vi "AFscanFineRange.vi"(8 "error in (no error)":errorcluster, 9 "ImageIn":T1, 10 "Session In":T2, 11 "controller in":refnum<k24>) -> (0 "error out":errorcluster, 1 "Image Out":T1, 2 "Session Out":T2, 3 "controller out":refnum<k24>, 4 "MaxVal":dbl, 5 "BestZ":dbl)   [LabVIEW 2019]
uses:
  C:/Users/TTUHEP/Documents/LabVIEW/Other Models/2010/Bin/Aerotech.A3200.dll
  Other Models/2010/Bin/Aerotech.A3200.dll
  <vilib>/vision/Image Controls.llb/IMAQ Image.ctl
  <vilib>/userDefined/High Color/IMAQdx.ctl
  <vilib>/vision/NI_Vision_Development_Module.lvlib
  <vilib>/vision/driver/NI_Vision_Acquisition_Software.lvlib
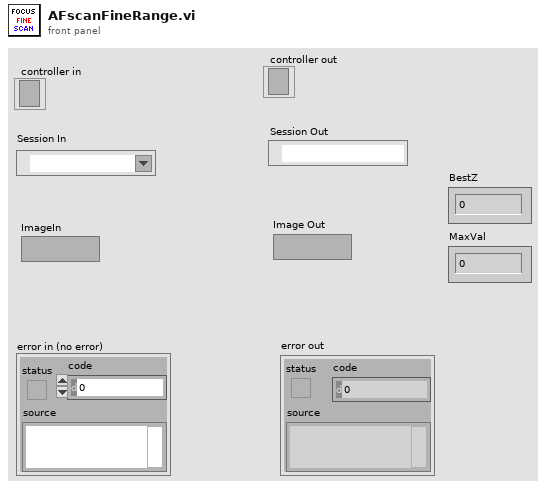
[diagram p1: front panel]
types:
  T1 = typedef "IMAQ Image.ctl" = refnum<image>
  T2 = typedef "IMAQdx.ctl" = refnum<k21>
  T3 = enum32{"Differentiation", "Gradient", "Prewitt", "Roberts", "Sigma", "Sobel"}
  T4 = typedef "Image Type" = u32
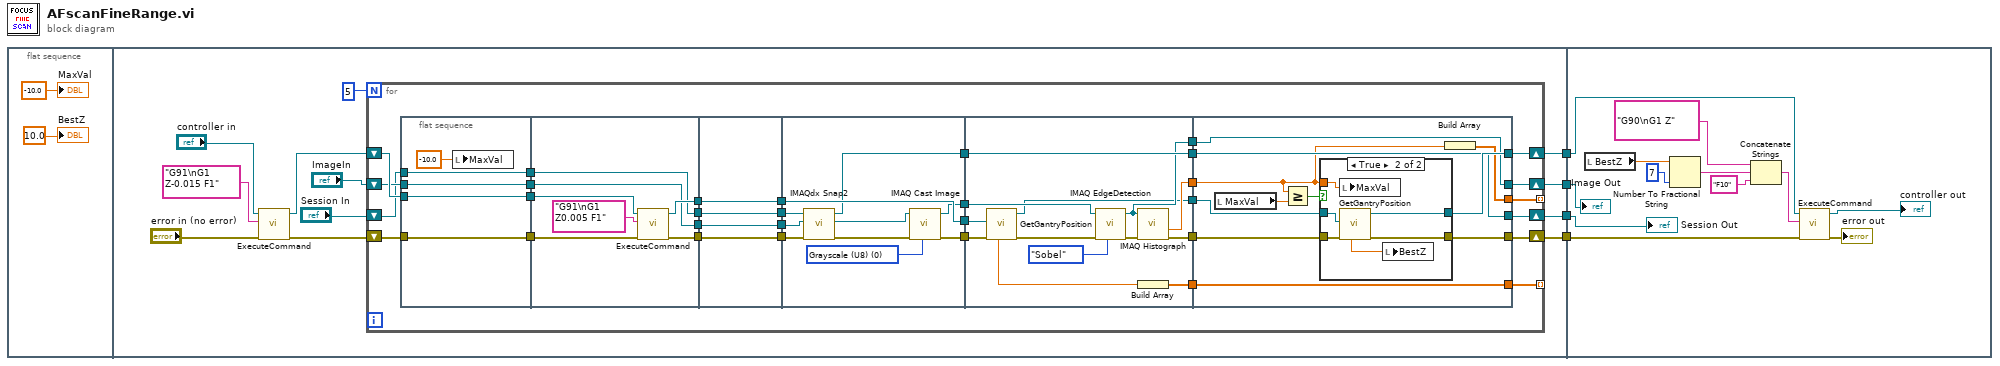
[diagram p0: block diagram]
diagram:
  n1 = flat-sequence {
    tunnel: [w13] -> w4
    tunnel: [w12] -> w3
    tunnel: [w8] -> w2
    tunnel: [w7] -> w1
    tunnel: w4 -> [w114]
    tunnel: w3 -> [w113]
    tunnel: w2 -> [w110]
    tunnel: w1 -> [w109]
    frame #0 {
      "BestZ" <- 10.0 ("BestZ")
      "MaxVal" <- -10.0 ("MaxVal")
    }
    frame #1 {
      n2 = call "ExecuteCommand.vi"("error in (no error)"="error in (no error)", "Command Code"="G91\nG1 Z-0.015 F1", "controller in"="controller in") -> ("error out"=w16:errorcluster, "controller out"=w17:refnum<k24>)  [unwired: 6 in, 1 out]
      n3 = for {
        N: 5 -> [_]
        shift-right: [w40] -> w8
        shift-left: "Session In" -> [w27]
        shift-right: [w41] -> w13
        shift-left: w16 -> [w50]
        shift-right: [w42] -> w12
        shift-left: w17 -> [w49]
        shift-right: [w29] -> w7
        shift-left: "ImageIn" -> [w33]
        tunnel: [w25] -> _ mode=indexing
        tunnel: [w24] -> _ mode=indexing
        n4 = flat-sequence {
          tunnel: [w55] -> w22
          tunnel: [w54] -> w21
          tunnel: [w53] -> w20
          tunnel: [w52] -> w19
          tunnel: w50 -> [w55]
          tunnel: w49 -> [w54]
          tunnel: w33 -> [w53]
          tunnel: w27 -> [w52]
          tunnel: [w61] -> w37
          tunnel: [w60] -> w35
          tunnel: [w57] -> w31
          tunnel: [w56] -> w28
          tunnel: w22 -> [w59]
          tunnel: w21 -> [w58]
          tunnel: w20 -> [w57]
          tunnel: w19 -> [w56]
          tunnel: w37 -> [w66]
          tunnel: [w66] -> w36
          tunnel: w35 -> [w65]
          tunnel: [w65] -> w34
          tunnel: [w64] -> w32
          tunnel: w31 -> [w64]
          tunnel: w28 -> [w63]
          tunnel: [w63] -> w26
          tunnel: w36 -> [w75]
          tunnel: w34 -> [w76]
          tunnel: [w76] -> w48
          tunnel: [w71] -> w47
          tunnel: [w70] -> w46
          tunnel: [w69] -> w38
          tunnel: w32 -> [w68]
          tunnel: w26 -> [w67]
          tunnel: w48 -> [w80]
          tunnel: w47 -> [w78]
          tunnel: w46 -> [w87]
          tunnel: [w79] -> w45
          tunnel: [w86] -> w44
          tunnel: [w85] -> w43
          tunnel: [w84] -> w39
          tunnel: w38 -> [w84]
          tunnel: [w83] -> w30
          tunnel: [w82] -> w23
          tunnel: w45 -> [w98]
          tunnel: w44 -> [w97]
          tunnel: w43 -> [w92]
          tunnel: [w96] -> w42
          tunnel: [w95] -> w41
          tunnel: [w94] -> w40
          tunnel: w39 -> [w94]
          tunnel: w30 -> [w93]
          tunnel: [w93] -> w29
          tunnel: [w91] -> w25
          tunnel: [w90] -> w24
          tunnel: w23 -> [w91]
          frame #0 {
            n5 = local write "MaxVal"(-10.0) -> ()
          }
          frame #1 {
            n6 = call "ExecuteCommand.vi"("error in (no error)"=w59, "Command Code"="G91\nG1 Z0.005 F1", "controller in"=w58) -> ("error out"=w61:errorcluster, "controller out"=w60:refnum<k24>)  [unwired: 6 in, 1 out]
          }
          frame #2 {
          }
          frame #3 {
            w74 = T4 0 items=["Grayscale (U8)", "Grayscale (I16)", "Grayscale (SGL)", "Complex (CSG)", "RGB (U32)", "HSL (U32)", "RGB (U64)", "Grayscale (U16)"] ("Image Type")
            n7 = call <vilib>:"IMAQdx Snap2.vi"("error in"=w75, "Image In"=w68, "Session In"=w67) -> ("error out"=w73:errorcluster, "Image Out"=w72:T1, "Session Out"=w69:T2)  [unwired: 6 in]
            n8 = call "IMAQ Cast Image"("Image Type"=w74, "error in (no error)"=w73, "Image Src"=w72) -> ("error out"=w71:errorcluster, "Image Dst Out"=w70:T1)  [unwired: 7 in]
          }
          frame #4 {
            n9 = call "GetGantryPosition.vi"("error in (no error)"=w78, "Controller In"=w80) -> ("error out"=w77:errorcluster, "controller out"=w79:refnum<k24>, "Position Z"=w81:dbl)  [unwired: 3 in, 4 out]
            n10 = call "IMAQ EdgeDetection"("Method"=T3."Sobel", "error in (no error)"=w77, "Image Src"=w87) -> ("error out"=w89:errorcluster, "Image Dst Out"=w83:T1)  [unwired: 7 in]
            n11 = call "IMAQ Histograph"("error in (no error)"=w89, "Image"=w83) -> ("error out"=w86:errorcluster, "Standard  Deviation"=w85:sgl)  [unwired: 6 in, 2 out]
            n12 = Build Array(w81) -> (w82:dbl[])
          }
          frame #5 {
            n13 = local read "MaxVal"() -> (w100:dbl)
            n14 = Greater Or Equal?(x=w92, y=w100) -> (x >= y?=w99:bool)
            n15 = case shown="True" w99 {
              tunnel: w92 -> [_ w103]
              tunnel: w98 -> [w101 w108]
              tunnel: [w101 w105] -> w96
              tunnel: w97 -> [w102 w107]
              tunnel: [w102 w106] -> w95
              frame False {
              }
              frame True {
                n16 = local write "MaxVal"(w103) -> ()
                n17 = call "GetGantryPosition.vi"("error in (no error)"=w107, "Controller In"=w108) -> ("error out"=w106:errorcluster, "controller out"=w105:refnum<k24>, "Position Z"=w104:dbl)  [unwired: 3 in, 4 out]
                n18 = local write "BestZ"(w104) -> ()
              }
            }
            n19 = Build Array(w92) -> (w90:sgl[])
          }
        }
      }
    }
    frame #2 {
      n20 = local read "BestZ"() -> (w120:dbl)
      n21 = Number To Fractional String(number=w120, precision (6)=i16 7) -> (F-format string=w118:string)  [unwired: 2 in]
      n22 = Concatenate Strings("G90\nG1 Z", w118, "F10" ("string")) -> (w119:string)
      n23 = call "ExecuteCommand.vi"("error in (no error)"=w114, "Command Code"=w119, "controller in"=w113) -> ("error out"=→"error out":errorcluster, "controller out"=→"controller out":refnum<k24>)  [unwired: 6 in, 1 out]
      "Session Out" <- w110
      "Image Out" <- w109
    }
  }
